vi "Test Unnamed Clusters to JSON Arrays.vi"() -> ()   [LabVIEW 2013]
uses:
  JSONtext.lvlib
panel:
  out "<JSON>":string
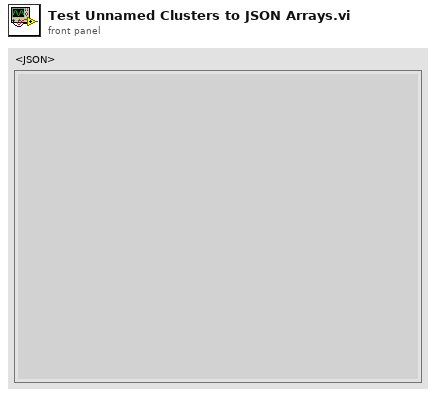
[diagram p1: front panel]
types:
  T1 = cluster{cluster{string, "<JSON>":string, i32}, cluster{"Name":string, "<JSON>Config":string}[]}
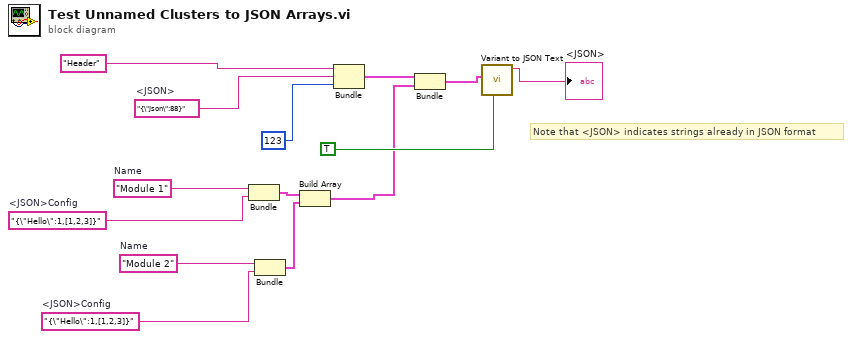
[diagram p0: block diagram]
diagram:
  w5 = "{\"Hello\":1,[1,2,3]}"  # <JSON>Config
  w6 = "{\"Hello\":1,[1,2,3]}"  # <JSON>Config
  w7 = "Module 2"  # Name
  w8 = "Module 1"  # Name
  w10 = "{\"Json\":88}"  # <JSON>
  # "Note that <JSON> indicates strings already in JSON format"
  n1 = Bundle("Name"=w8, "<JSON>Config"=w5) -> (w9:cluster{"Name":string, "<JSON>Config":string})  [unwired: 1 in]
  n2 = Bundle("Name"=w7, "<JSON>Config"=w6) -> (w4:cluster{"Name":string, "<JSON>Config":string})  [unwired: 1 in]
  n3 = Build Array(w9, w4) -> (w2:cluster{"Name":string, "<JSON>Config":string}[])
  n4 = Bundle("Header", "<JSON>"=w10, 123) -> (w14:cluster{string, "<JSON>":string, i32})  [unwired: 1 in]
  n5 = Bundle(w14, w2) -> (w13:T1)  [unwired: 1 in]
  n6 = call "Variant to JSON Text.vi"("Pretty Print?"=TRUE, "Variant"=w13) -> ("<JSON>"=→"<JSON>":string)  [unwired: 8 in, 1 out]
